vi "Get Methods.vi"(8 "error in (no error)":errorcluster, 11 "Node in":refnum<class "CallHandler.lvclass">) -> (0 "error out":errorcluster, 2 "Method List (Enum or Str Array)":variant, 3 "Node out":refnum<class "CallHandler.lvclass">)   [LabVIEW 2013, in "JKI_Python_Bridge_for_LV.lvlib" / "CallHandler.lvclass"]
uses:
  CallHandler.lvclass
  CallHandler.lvclass/CallHandler.ctl
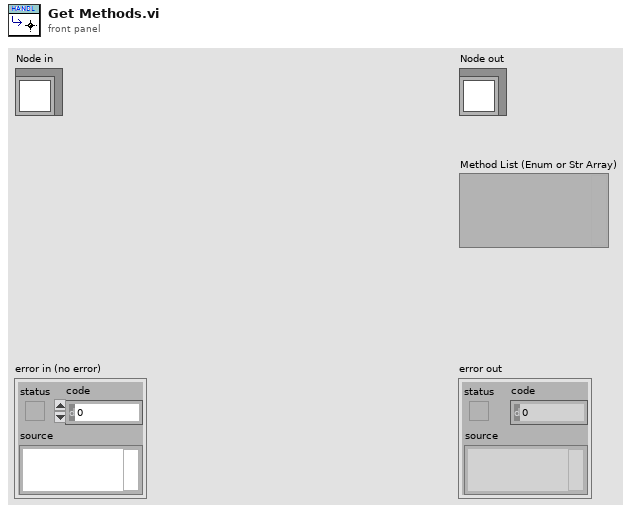
[diagram p1: front panel]
types:
  T1 = typedef "JKI_Python_Bridge_for_LV.lvlib/CallHandler.lvclass/Private Data.ctl" = cluster{"Call Registration":T2, "Method List (VEnum)":variant, "Object Name":string}
  T2 = typedef "JKI_Python_Bridge_for_LV.lvlib/Server.lvclass/Python Method Call - Event Registration.ctl" = refnum<event-registration>
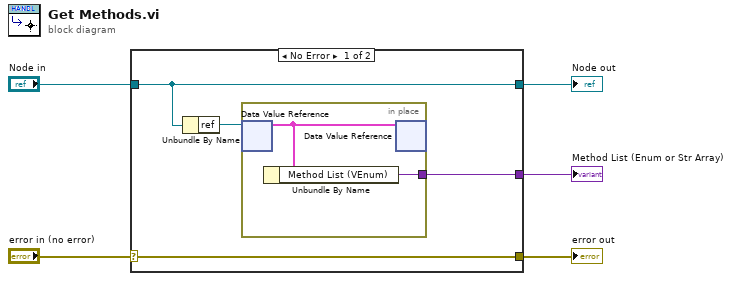
[diagram p0: block diagram]
diagram:
  n1 = case shown="No Error" "error in (no error)" {
    selector: "error in (no error)" -> [w9 w12]
    tunnel: [w9 w12] -> w4
    tunnel: [w8 w13] -> w2
    tunnel: "Node in" -> [w8 w13]
    tunnel: [w6 _] -> w1
    frame No Error {
      n2 = Unbundle By Name(w8) -> ("ref"=w7:refnum<data-value>)
      n3 = in-place {
        in-place-border: [w10] -> w6
        n4 = in-place-dvr #1(w7) -> (w11:T1)  [unwired: 1 out]
        n5 = Unbundle By Name(w11) -> ("Method List (VEnum)"=w10:variant)
        n6 = in-place-dvr #1(w11) -> ()  [unwired: 2 out]
      }
    }
    frame Error {
    }
  }
  "error out" <- w4
  "Node out" <- w2
  "Method List (Enum or Str Array)" <- w1
